vi "Open Audio File Read (Polymorphic Template).vi"   [LabVIEW 2020]
uses:
  Private/Result To Error.vi
  11be0b8a-0ecf-48c6-ad13-a826563776bf.vi/56465d8a-8d83-4810-9820-5ab2fa709974.vi
  4eec47c5-3867-48fc-af9a-773a85a8cbd4.vi/56465d8a-8d83-4810-9820-5ab2fa709974.vi
  <vilib>/Utility/error.llb/Error Cluster From Error Code.vi
  ed691427-ca1e-430d-8efd-443bc37f0ad6.vi
  dc509e6d-59c1-4a7a-bac3-014c3c6b5a28.vi
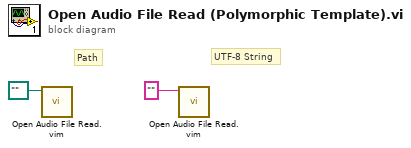
[diagram p0: block diagram]
diagram:
  # "UTF-8 String"
  # "Path"
  n1 = call "Open Audio File Read.vim"("Path"=path "" ("Path In")) -> ()  [unwired: 9 in, 2 out]
  n2 = call "Open Audio File Read.vim"("Path"="") -> ()  [unwired: 9 in, 2 out]
